vi "Send Force Sensor Notification.vi"(8 "error in (no error)":errorcluster, 10 "fs notifier":refnum<notifier>, 11 "Force Sensor in":refnum<class "Force Sensor.lvclass">) -> (0 "error out":errorcluster)   [LabVIEW 2020]
uses:
  Sensors/Force Sensors/Force Sensor.lvclass
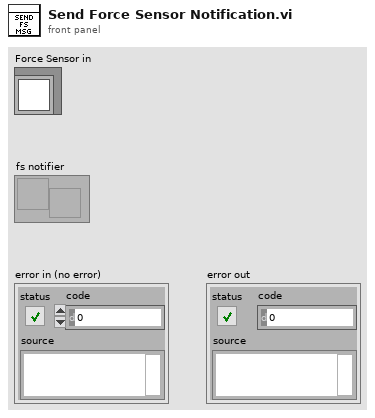
[diagram p1: front panel]
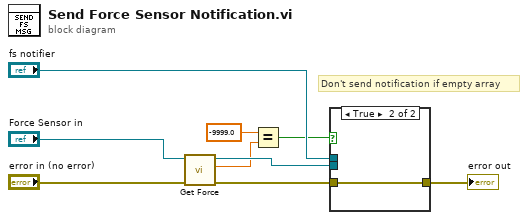
[diagram p0: block diagram]
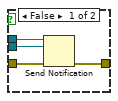
[diagram p2: hidden frame]
diagram:
  # "Don't send notification if empty array"
  n1 = call "Get Force.vi"("error in (no error)"="error in (no error)", "Force Sensor in"="Force Sensor in") -> ("error out"=w4:errorcluster, "force (V)"=w3:dbl, "Force Sensor out"=w6:refnum<class "Force Sensor.lvclass">)  [unwired: 7 in]
  n2 = Equal?(x=-9999.0, y=w3) -> (x = y?=w1:bool)
  n3 = case shown="True" w1 {
    tunnel: "fs notifier" -> [w13 _]
    tunnel: [w12 w14] -> w8
    tunnel: w6 -> [w11 _]
    tunnel: w4 -> [w10 w14]
    frame False {
      n4 = Send Notification(notification=w11, notifier=w13, error in (no error)=w10) -> (error out=w12:errorcluster)  [unwired: 1 out]
    }
    frame True {
    }
  }
  "error out" <- w8
